vi "DataFilter_Logging.vi"(10 "Input Array":dbl[](array[numeric]), 11 "rt fifo":refnum<k33>) -> (3 "rt fifo out":refnum<k33>)   [LabVIEW 2020]
panel:
  out "error out":errorcluster
  out "# elements":u32
  out "Array 2":dbl[][](array[numeric])
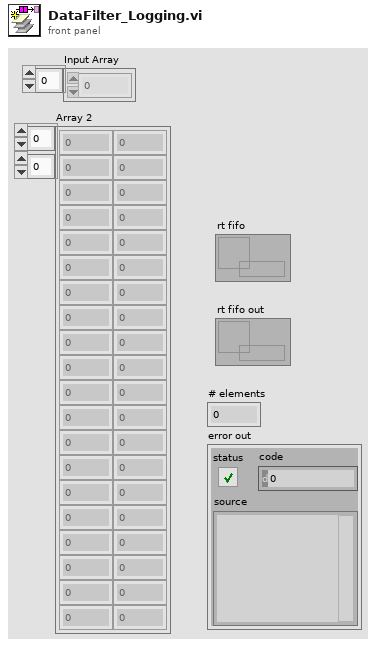
[diagram p1: front panel]
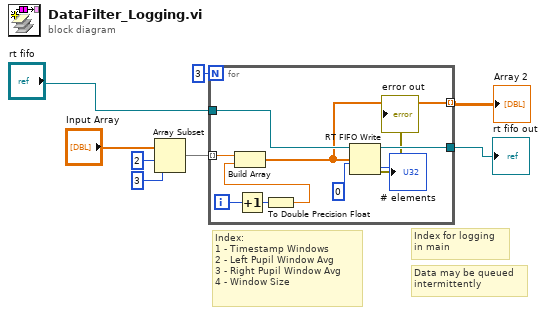
[diagram p0: block diagram]
diagram:
  # "Data may be queued \nintermittently"
  # "Index for logging \nin main"
  # "Index: \n1 - Timestamp Windows \n2 - Left Pupil Window Avg \n3 - Right Pupil Window Avg\n4 - Window Size"
  n1 = Array Subset(array="Input Array", index=2, length=3) -> (w8:dbl[])
  n2 = for {
    N: 3 -> [_]
    tunnel: w8 -> [w18] mode=indexing
    tunnel: "rt fifo" -> [w16]
    tunnel: [w15] -> w1
    tunnel: [w14] -> w2 mode=indexing
    i -> [w13]
    n3 = Increment(x=w13) -> (x+1=w12:i32)
    n4 = To Double Precision Float(number=w12) -> (double precision float=w17:dbl)
    n5 = Build Array(w18, w17) -> (w14:dbl[])
    n6 = RT FIFO Write(0:w16, 1:w14, 2:0 ("timeout in ms (0)")) -> (7:→"# elements":u32, 8:w15:refnum<k33>, 11:→"error out":errorcluster)  [unwired: 2 in, 1 out]
  }
  "Array 2" <- w2
  "rt fifo out" <- w1
